vi "18-ReplaceLeftExplode.vi"(10 "Left Explosion":u64, 11 "Left Snailfish Number in":string) -> (3 "Left Snailfish Number out":string)   [LabVIEW 2019, in "18.lvlib"]
uses:
  18.lvlib
  <vilib>/regexp/Match Regular Expression.xnode
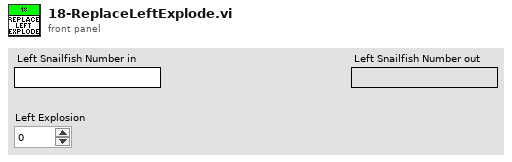
[diagram p1: front panel]
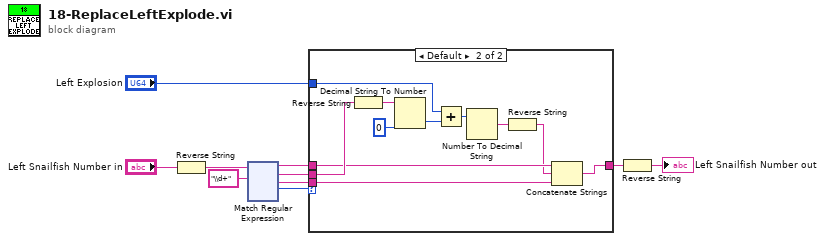
[diagram p0: block diagram]
diagram:
  n1 = Reverse String(1:"Left Snailfish Number in") -> (0:w7:string)
  n2 = xnode "Match Regular Expression"("input string"=w7, "regular expression"="\\d+") -> ("before match"=w5:string, "whole match"=w3:string, "after match"=w4:string, "offset past match"=w6:i32)  [unwired: 4 in, 1 out]
  n3 = case shown="Default" w6 {
    tunnel: "Left Explosion" -> [_ w21]
    tunnel: w5 -> [w11 w15]
    tunnel: w4 -> [_ w13]
    tunnel: w3 -> [_ w18]
    tunnel: [w11 w12] -> w1
    frame -1 {
    }
    frame Default {
      n4 = Reverse String(1:w18) -> (0:w17:string)
      n5 = Decimal String To Number(string=w17, default (0L)=u64 0 ("default (0 I32)")) -> (number=w22:u64)  [unwired: 1 in, 1 out]
      n6 = Add(x=w21, y=w22) -> (x+y=w19:u64)
      n7 = Number To Decimal String(number=w19) -> (decimal integer string=w16:string)  [unwired: 1 in]
      n8 = Reverse String(1:w16) -> (0:w14:string)
      n9 = Concatenate Strings(w15, w14, w13) -> (w12:string)
    }
  }
  n10 = Reverse String(1:w1) -> (0:→"Left Snailfish Number out":string)
